vi "Demo - Simple Use Testing.vi"() -> ()   [LabVIEW 2013]
uses:
  Private/Get Variable - polymorph parts/Get String.vi
  Private/Get Variable - polymorph parts/Get Double.vi
  Private/Get Variable - polymorph parts/Get Double Complex.vi
  Private/Get Variable - polymorph parts/Get 1D Array Double.vi
  Private/Get Variable - polymorph parts/Get 1D Array String.vi
  Private/Get Variable - polymorph parts/Get 1D Array Double Complex.vi
  Private/Get Variable - polymorph parts/Get 2D Array Double.vi
  Private/Get Variable - polymorph parts/Get 2D Array Double Complex.vi
  GOLPI library.lvlib
panel:
  in  "data type array 5":cdb[][](array[numeric])
  in  "data type array 4":dbl[][](array[numeric])
  in  "use temporary file?":bool
  in  "data type array 3":cdb[](array[numeric])
  in  "data type array 2":string[](array[string])
  in  "data type 4":cdb
  in  "data type 3":dbl
  in  "Get variable":T1(tab)=enum."vector strings"
  out "s":string
  out "r":dbl format="%.2f"
  out "c":cdb format="%.2f"
  out "vs length":i32
  out "vs":string[](array[string])
  out "vr":dbl[](array[numeric])
  out "vr length":i32
  out "vc length":i32
  out "vc":cdb[](array[numeric])
  out "mr":dbl[][](array[numeric]) format="%.2f"
  out "mr sizes":i32[](array[numeric])
  out "mc sizes":i32[](array[numeric])
  out "mc":cdb[][](array[numeric]) format="%.2f"
  in  "data type array":dbl[](array[numeric])
  in  "data type":string
  in  "variable name":string="x"
  in  "command":string="x=[1 2 3]\ndisp('OK')"
  out "GNU Octave version":string
  out "exit code":i32
  out "error out":errorcluster
  out "read buffer":string
  in  "Octave binary directory":path=path "C:/Program Files/Octave-3.6.2/bin"
  in  "Working directory":path=path "C:/"
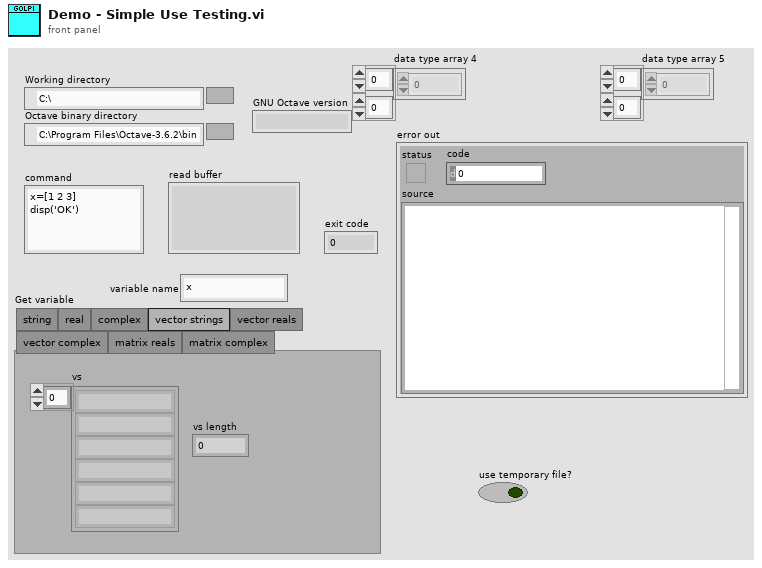
[diagram p1: front panel]
types:
  T1 = enum32{"string", "real", "complex", "vector strings", "vector reals", "vector complex", "matrix reals", "matrix complex"}
  T2 = typedef "GOLPI library.lvlib/GOLPI reference Type Def.ctl" = cluster{"pipe handle":T3, "fast read timeout [ms]":u32, "fast read settle time [ms]":u32, "fast read to multiple [ms]":u32, "max elements per input line":u32, "slow read timeout [ms]":u32}
  T3 = typedef "LV Process.lvlibp/Pipe Handle.ctl" = cluster{"lv_proc.dll file path":path, "process instance handle":u32[]}
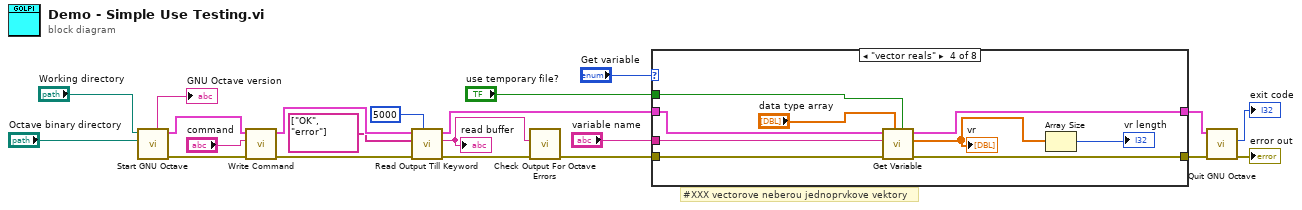
[diagram p0: block diagram]
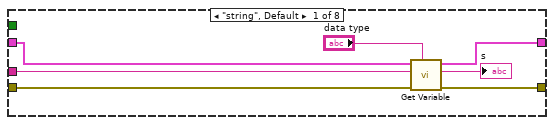
[diagram p2: hidden frame]
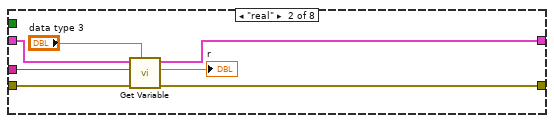
[diagram p3: hidden frame]
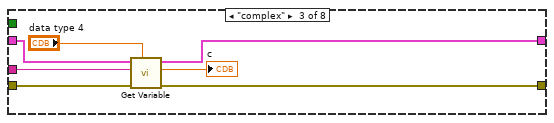
[diagram p4: hidden frame]
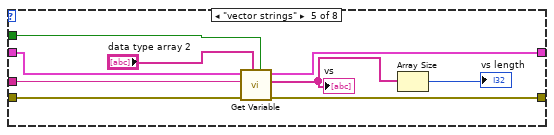
[diagram p5: hidden frame]
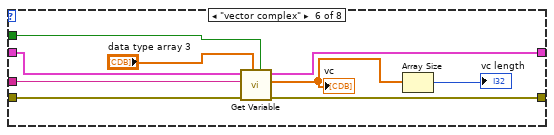
[diagram p6: hidden frame]
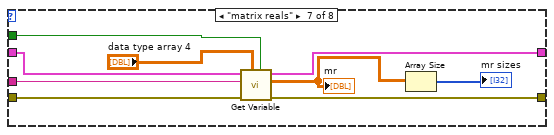
[diagram p7: hidden frame]
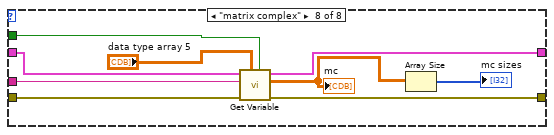
[diagram p8: hidden frame]
diagram:
  # "#XXX vectorove neberou jednoprvkove vektory"
  n1 = call "Start GNU Octave.vi"("Octave binary directory"="Octave binary directory", "Working directory"="Working directory") -> ("error out"=w17:errorcluster, "GOLPI ref. out"=w19:T2, "GNU Octave version"=→"GNU Octave version":string)  [unwired: 6 in, 1 out]
  n2 = call "Write Command.vi"("error in"=w17, "command"="command", "GOLPI ref. in"=w19) -> ("error out"=w16:errorcluster, "GOLPI ref. out"=w18:T2)  [unwired: 7 in]
  n3 = call "Read Output Till Keyword.vi"("timeout [ms]"=u32 5000, "error in"=w16, "keywords"=string[] ["OK", "error"], "GOLPI ref. in"=w18) -> ("error out"=w9:errorcluster, "read buffer"=w7:string, "GOLPI ref. out"=w13:T2)  [unwired: 4 in, 1 out]
  "read buffer" <- w7
  n4 = call "Check Output For Octave Errors.vi"("error in"=w9, "read buffer"=w7) -> ("error out"=w8:errorcluster)  [unwired: 9 in]
  n5 = case shown="\"vector reals\"" "Get variable" {
    tunnel: w13 -> [w27 w32 w40 w49 w57 w65 w77 w86]
    tunnel: [w24 w30 w37 w48 w54 w62 w73 w83] -> w12
    tunnel: [w25 w29 w36 w47 w55 w63 w74 w82] -> w11
    tunnel: "variable name" -> [w22 w33 w38 w50 w58 w66 w76 w84]
    tunnel: w8 -> [w26 w34 w39 w51 w56 w64 w75 w85]
    tunnel: "use temporary file?" -> [_ _ _ w44 w52 w61 w71 w81]
    frame "string", Default {
      n6 = call-poly "Get Variable.vi"("data type of variable"="data type", "error in"=w26, "variable name"=w22, "GOLPI ref. in"=w27) -> ("error out"=w25:errorcluster, "value"=→"s":string, "GOLPI ref. out"=w24:T2)  [unwired: 5 in]
    }
    frame "real" {
      n7 = call-poly "Get Variable.vi"("data type of variable"="data type 3", "error in"=w34, "variable name"=w33, "GOLPI ref. in"=w32) -> ("error out"=w29:errorcluster, "value"=→"r":dbl, "GOLPI ref. out"=w30:T2)  [unwired: 5 in]
    }
    frame "complex" {
      n8 = call-poly "Get Variable.vi"("data type of variable"="data type 4", "error in"=w39, "variable name"=w38, "GOLPI ref. in"=w40) -> ("error out"=w36:errorcluster, "value"=→"c":cdb, "GOLPI ref. out"=w37:T2)  [unwired: 5 in]
    }
    frame "vector reals" {
      n9 = call-poly "Get Variable.vi"("use temporary file?"=w44, "data type of variable"="data type array", "error in"=w51, "variable name"=w50, "GOLPI ref. in"=w49) -> ("error out"=w47:errorcluster, "value"=w43:dbl[], "GOLPI ref. out"=w48:T2)  [unwired: 4 in]
      "vr" <- w43
      n10 = Array Size(array=w43) -> (size(s)=→"vr length":i32)
    }
    frame "vector strings" {
      n11 = call-poly "Get Variable.vi"("use temporary file?"=w52, "data type of variable"="data type array 2", "error in"=w56, "variable name"=w58, "GOLPI ref. in"=w57) -> ("error out"=w55:errorcluster, "value"=w53:string[], "GOLPI ref. out"=w54:T2)  [unwired: 4 in]
      "vs" <- w53
      n12 = Array Size(array=w53) -> (size(s)=→"vs length":i32)
    }
    frame "vector complex" {
      n13 = call-poly "Get Variable.vi"("use temporary file?"=w61, "data type of variable"="data type array 3", "error in"=w64, "variable name"=w66, "GOLPI ref. in"=w65) -> ("error out"=w63:errorcluster, "value"=w67:cdb[], "GOLPI ref. out"=w62:T2)  [unwired: 4 in]
      "vc" <- w67
      n14 = Array Size(array=w67) -> (size(s)=→"vc length":i32)
    }
    frame "matrix reals" {
      n15 = call-poly "Get Variable.vi"("use temporary file?"=w71, "data type of variable"="data type array 4", "error in"=w75, "variable name"=w76, "GOLPI ref. in"=w77) -> ("error out"=w74:errorcluster, "value"=w70:dbl[][], "GOLPI ref. out"=w73:T2)  [unwired: 4 in]
      "mr" <- w70
      n16 = Array Size(array=w70) -> (size(s)=→"mr sizes":i32[])
    }
    frame "matrix complex" {
      n17 = call-poly "Get Variable.vi"("use temporary file?"=w81, "data type of variable"="data type array 5", "error in"=w85, "variable name"=w84, "GOLPI ref. in"=w86) -> ("error out"=w82:errorcluster, "value"=w79:cdb[][], "GOLPI ref. out"=w83:T2)  [unwired: 4 in]
      "mc" <- w79
      n18 = Array Size(array=w79) -> (size(s)=→"mc sizes":i32[])
    }
  }
  n19 = call "Quit GNU Octave.vi"("error in"=w11, "GOLPI ref. in"=w12) -> ("error out"=→"error out":errorcluster, "exit code"=→"exit code":i32)  [unwired: 8 in]
